vi "Test Worker Job Count Incremented.vi"(8 "error in (no error)":errorcluster, 11 "Barista Test in":refnum<class "Barista Test.lvclass">) -> (0 "error out":errorcluster, 3 "Barista Test out":refnum<class "Barista Test.lvclass">)   [LabVIEW 2020, in "Barista Test.lvclass"]
uses:
  Barista Test.lvclass
  C:/git/astemes-triarc-examples/source/Coffee Shop/Tests/Worker Test/Worker Test.lvclass
  C:/Program Files (x86)/National Instruments/LabVIEW 2020/vi.lib/Astemes/LUnit/Test Case.lvclass
  Test Doubles/Stub Job Handler/Stub Job Handler.lvclass
  C:/git/astemes-triarc-examples/source/Coffee Shop/Processes/People/Process Job/Job Handler.lvclass
  Support/Beverages/Beverage/Beverage.lvclass
  <vilib>/Astemes/Triarc Framework/Process/Process.lvclass/Process.ctl
  <vilib>/Astemes/LUnit/Test Case.lvclass/Test Case.ctl
  <vilib>/Astemes/Triarc Framework/Process/Public/Lifecycle/Get Lifecycle State.vi
  <vilib>/Astemes/Triarc Framework/Support/Execution timer.vi
  <vilib>/Astemes/Triarc Framework/Process/Private/SubVIs/Wait for finish.vi
  <vilib>/Astemes/Triarc Framework/Process/Private/SubVIs/Set Lifecycle State.vi
  <vilib>/Astemes/Triarc Framework/Process/Protected/Messaging/Send Message.vi
  <vilib>/Astemes/LUnit/Palette/Pass If Equal.vi/cbf50e99-f124-4847-863a-8e9794d3dede.vi
  <vilib>/Utility/error.llb/Clear Errors.vi
  <vilib>/Astemes/Triarc Framework/Process/Private/SubVIs/Handle Debug Data.vi
  <vilib>/Astemes/LUnit/Append Pass Result.vi
  <vilib>/Astemes/LUnit/Append Fail Result.vi
  <vilib>/Astemes/LUnit/Describe Comparison.vi
  <vilib>/Astemes/LUnit/Compare Variants.vi
  <vilib>/Astemes/Triarc Framework/Logging/Log Debug.vi
  <vilib>/AdvancedString/1D String Array to Delimited String.vi
  <vilib>/Utility/High Resolution Relative Seconds.vi
  <vilib>/Astemes/LUnit/Variant to string.vi
  Processes/People/Workers/Worker/Worker.lvclass
  C:/Program Files (x86)/National Instruments/LabVIEW 2020/vi.lib/Astemes/Triarc Framework/Process/Process.lvclass
  <vilib>/Utility/error.llb/Error Cluster From Error Code.vi
  <vilib>/Astemes/Triarc Framework/Support/Dequeue Broadcast Message.vi
  <vilib>/Astemes/Triarc Framework/Process/Public/Read Name.vi
  <vilib>/Utility/Data Type/Get Type Information.vi
  <vilib>/Utility/LVClass/Get LV Class Name.vi
  <vilib>/Astemes/Triarc Framework/Callback/Callback.lvclass
  <vilib>/Astemes/Triarc Framework/Process/Process.lvclass
  Worker Test/Worker Test.lvclass
  <vilib>/Astemes/LUnit/Test Case.lvclass
  Support/Order Item/Order Item.lvclass
  <vilib>/Astemes/Triarc Framework/Support/Broadcast Event Dequeuers.lvlib
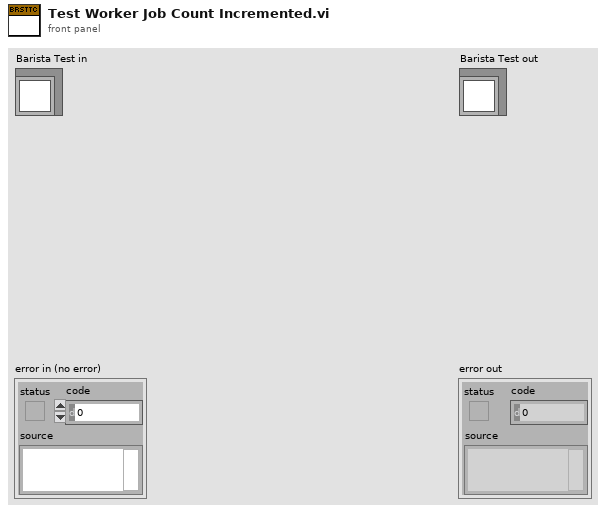
[diagram p1: front panel]
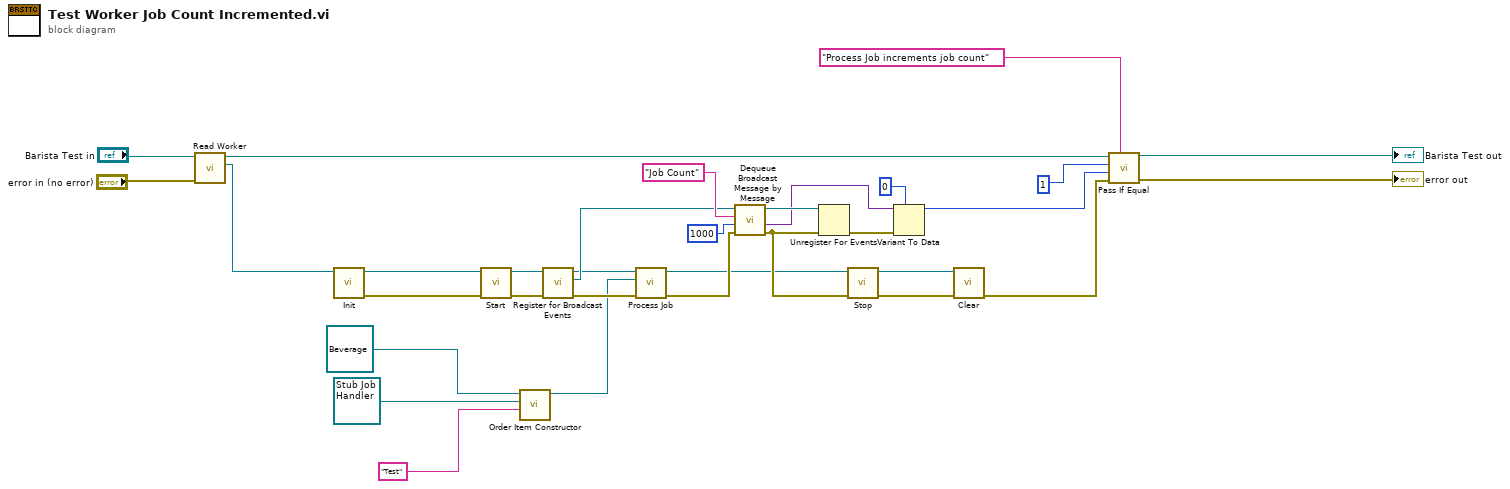
[diagram p0: block diagram]
diagram:
  n1 = call "Read Worker.vi"("error in (no error)"="error in (no error)", "Worker Test in"="Barista Test in") -> ("Worker"=w6:refnum<class "Worker.lvclass">, "Worker Test out"=w5:refnum<class "Barista Test.lvclass">)  [unwired: 7 in, 1 out]
  n2 = call-dynamic "Init.vi"("View In"=w6) -> ("error out"=w7:errorcluster, "View Out"=w10:refnum<class "Worker.lvclass">)  [unwired: 9 in]
  n3 = call <vilib>:"Start.vi"("error in (no error)"=w7, "Process In"=w10) -> ("error out"=w11:errorcluster, "Process Out"=w15:refnum<class "Worker.lvclass">)  [unwired: 7 in, 1 out]
  n4 = call "Order Item Constructor.vi"("Cust Name"="Test", "Pick Up Order Handler"=refnum<class "Stub Job Handler.lvclass"> refnum ("Stub Job Handler.lvclass"), "Beverage"=refnum<class "Beverage.lvclass"> refnum) -> ("Order Item"=w1:refnum<class "Order Item.lvclass">)  [unwired: 7 in, 1 out]
  n5 = call <vilib>:"Register for Broadcast Events.vi"("error in (no error)"=w11, "Process In"=w15) -> ("error out"=w14:errorcluster, "Event Registration Refnum Out"=w19:refnum<event-registration>, "Process Out"=w16:refnum<class "Worker.lvclass">)  [unwired: 7 in]
  n6 = call-dynamic "Process Job.vi"("error in (no error)"=w14, "Job"=w1, "Worker In"=w16) -> ("error out"=w18:errorcluster, "Worker Out"=w17:refnum<class "Worker.lvclass">)  [unwired: 7 in]
  n7 = call <vilib>:"Dequeue Broadcast Message by Message.vi"("error in (no error)"=w18, "Timeout (-1)"=1000, "Message"="Job Count", "Event Registration Refnum"=w19) -> ("error out"=w25:errorcluster, "Message Data"=w22:variant, "Event Registration Refnum Out"=w28:refnum<event-registration>)  [unwired: 3 in, 2 out]
  n8 = Unregister For Events(event registration refnum=w28, error in=w25) -> (error out=w27:errorcluster)
  n9 = call <vilib>:"Stop.vi"("error in (no error)"=w25, "Process In"=w17) -> ("error out"=w9:errorcluster, "Process Out"=w8:refnum<class "Worker.lvclass">)  [unwired: 7 in, 1 out]
  n10 = Variant To Data(error in=w27, type=u32 0 ("code"), Variant=w22) -> (data=w24:u32)  [unwired: 1 out]
  n11 = call-dynamic "Clear.vi"("error in (no error)"=w9, "View In"=w8) -> ("error out"=w12:errorcluster)  [unwired: 9 in]
  n12 = call <vilib>:"Pass If Equal.vi"("Description"="Process Job increments job count", "error in (no error)"=w12, "Actual"=w24, "Expected"=u32 1 ("code"), "LUnit Test Case In"=w5) -> ("error out"=→"error out":errorcluster, "LUnit Test Case Out"=→"Barista Test out":refnum<class "Barista Test.lvclass">)  [unwired: 5 in]
